vi "final result simple.vi"(4 "norm type":string="std norm", 6 "q":string="17O q", 9 "error in":errorcluster) -> (1 "error out":errorcluster)   [LabVIEW 2016]
uses:
  <vilib>/Analysis/baseanly.llb/Mean (DBL).vi
  <vilib>/Analysis/NI_AALBase.lvlib
panel:
  out "array w/ subset deleted 2":dbl[][](array[numeric])
  out "size(s)":i32
  out "array w/ subset deleted":dbl[][](array[numeric])
  out "Numeric 4":i32
  out "Numeric 3":i32
  out "Numeric 2":i32
  out "sqrt(x) 3":dbl
  out "sqrt(x) 2":dbl
  out "sqrt(x)":dbl
  out "Array 4":dbl[](array[numeric])
  out "Array 15":dbl[](array[numeric])
  out "Array 14":dbl[](array[numeric])
  out "sequence result header":string[](array[string])
  out "subarray 2":string[](array[string])
  in  "Final result header":string[](array[string])=["position", "holder", "sample name", "number of cycles", "user", "Total Run Time(min)", "final ratio", "error", "percent error"]
  out "Array 13":dbl[](array[numeric])
  out "Array 12":dbl[](array[numeric])
  out "Array 11":dbl[](array[numeric])
  out "Final Result 2":string[][](array[string])
  out "Array 8":dbl[](array[numeric])
  out "Array 7":dbl[](array[numeric])
  out "subarray":dbl[](array[numeric])
  out "Numeric":dbl
  out "Cycle data by seq":dbl[][][](array[numeric])
  out "appended array":dbl[](array[numeric])
  out "Array 3":string[][](array[string])
  out "Array 2":string[](array[string])
  out "Array":string[][](array[string])
  out "sequence  Result":dbl[][](array[numeric])
  out "Final result header 2":string[](array[string])
  out "Final Result":string[](array[string])
  out "cycle result header":string[](array[string])
  out "Array 5":dbl[](array[numeric])
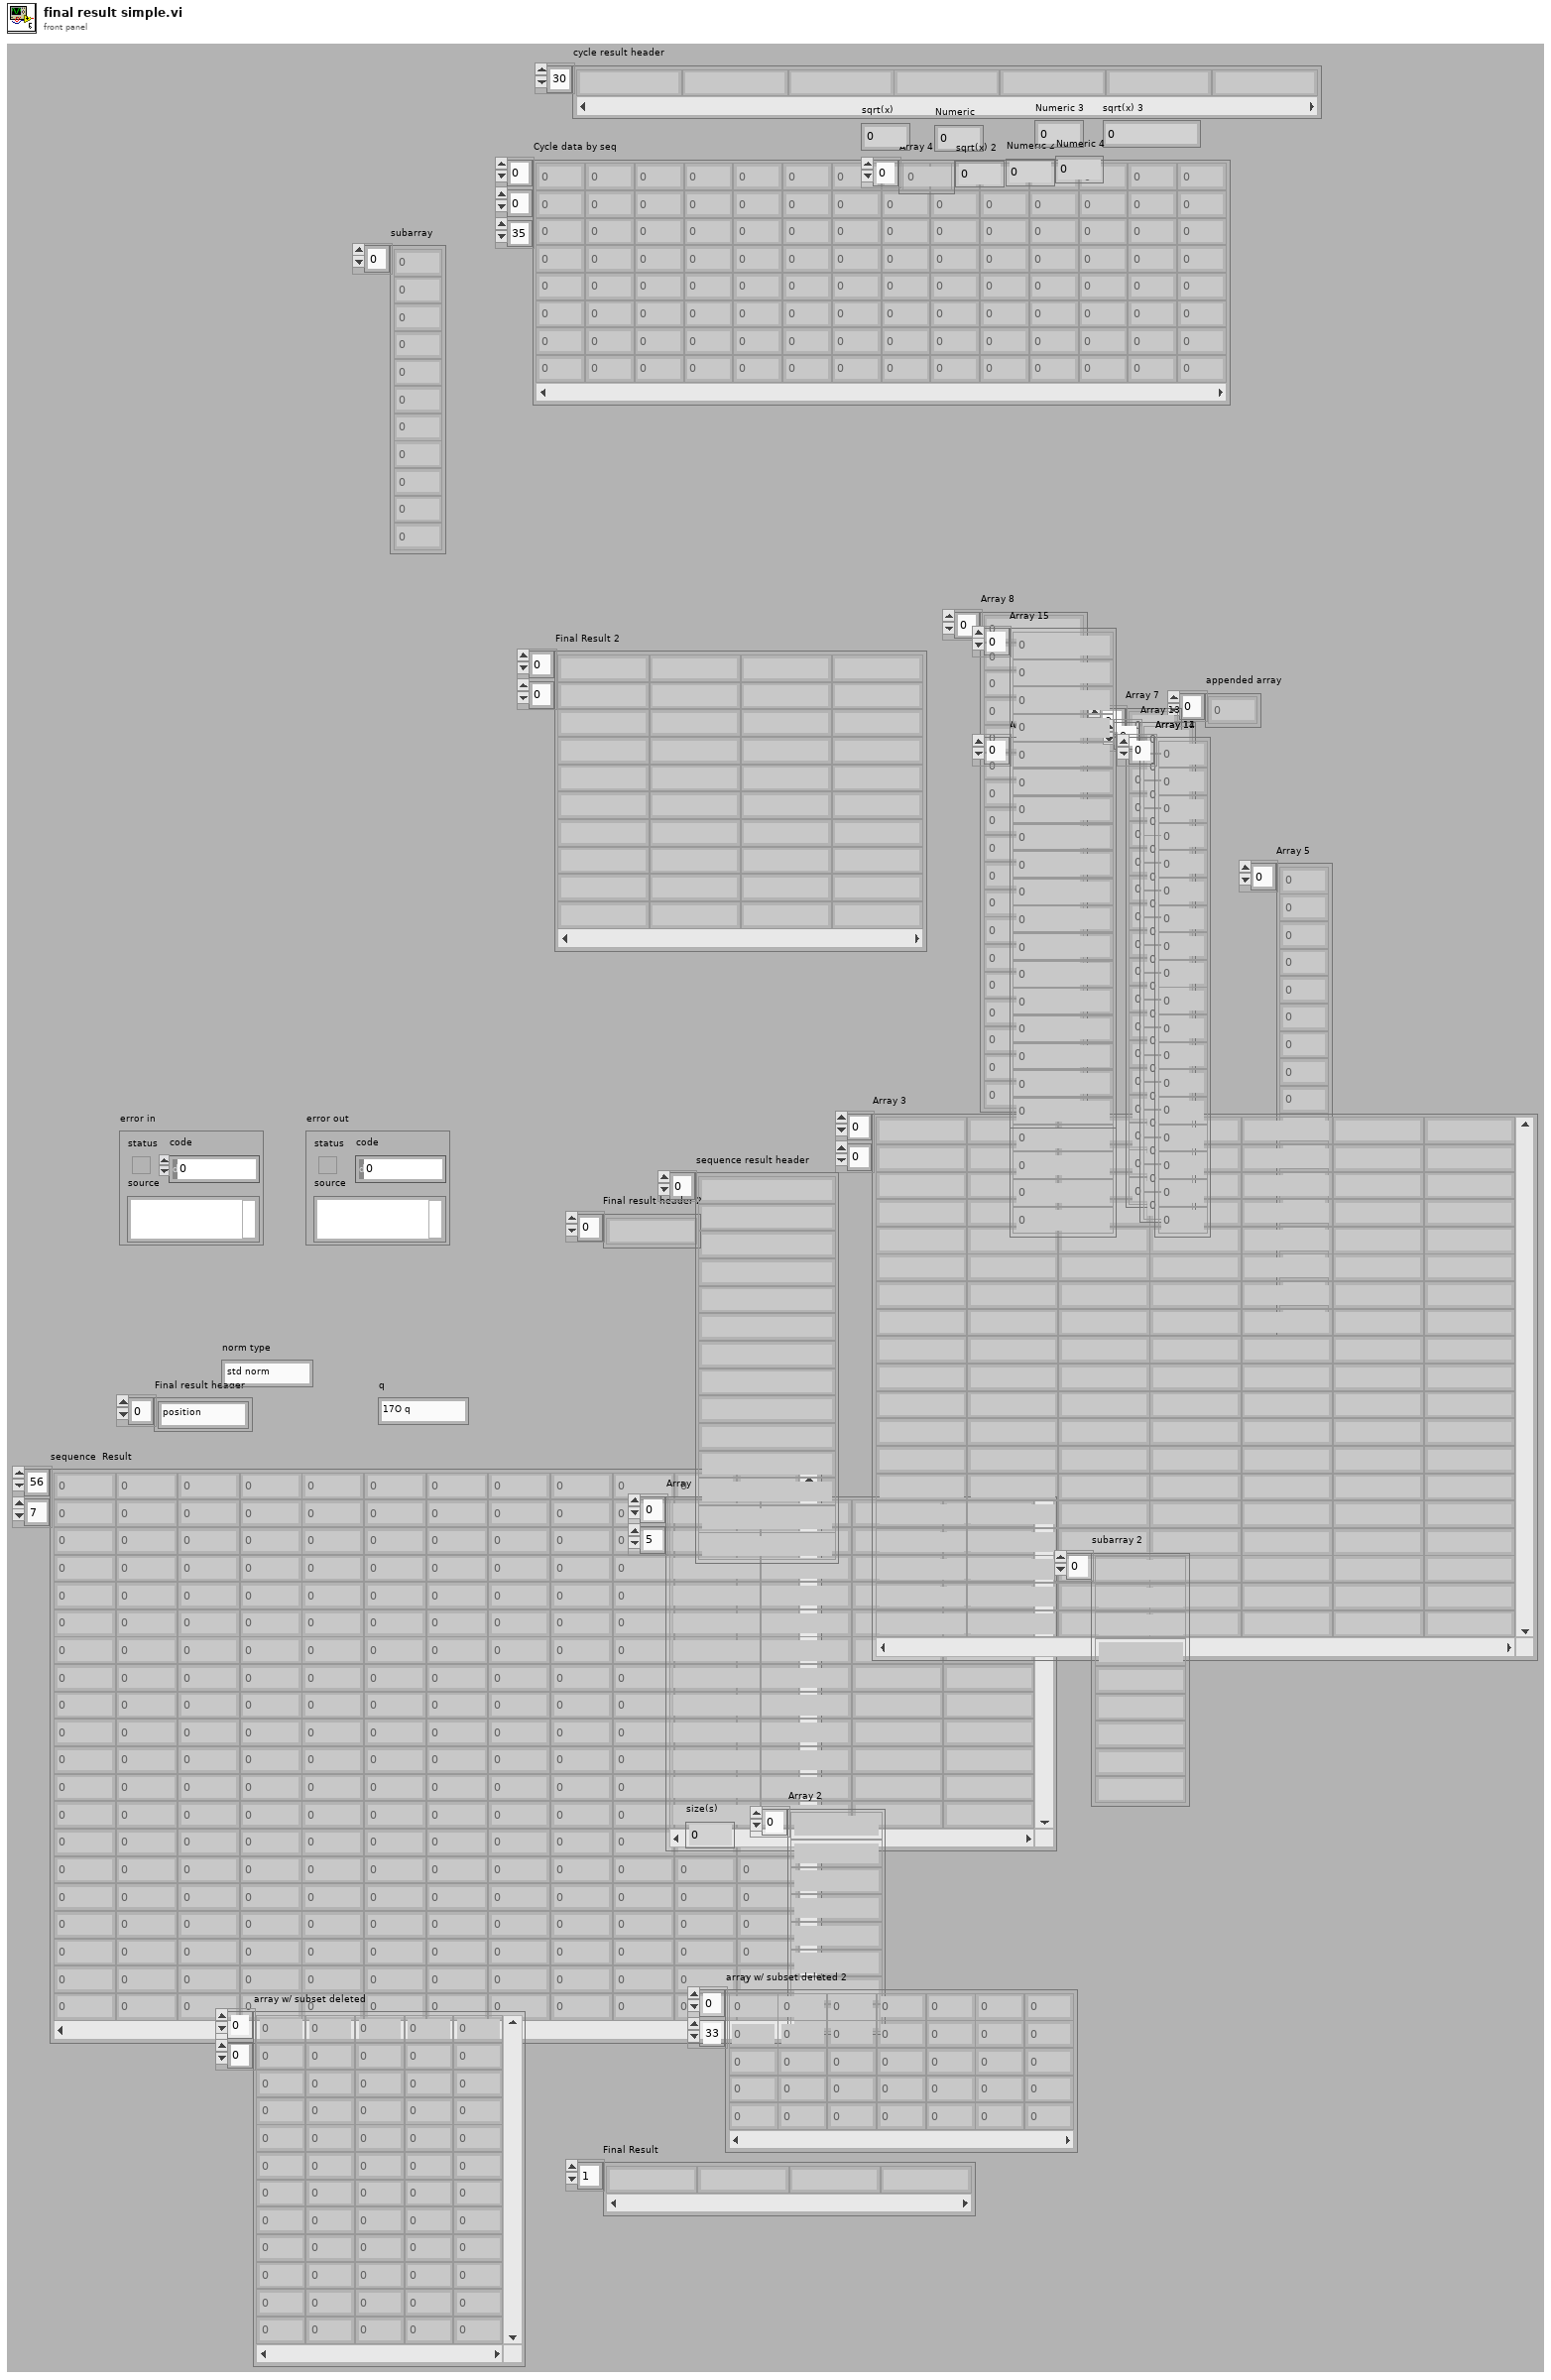
[diagram p1: front panel]
types:
  T1 = typedef "data control cluster.ctl" = cluster{"Final result header":string[], "sequence result header":string[], "cycle result header ":string[], "Final Result":string[][], "sequence  Result":dbl[][], "Cycle data by seq":dbl[][][], "Cycle data by position":dbl[][][], "Final seq  Result":dbl[][], "only specific type":dbl[][]}
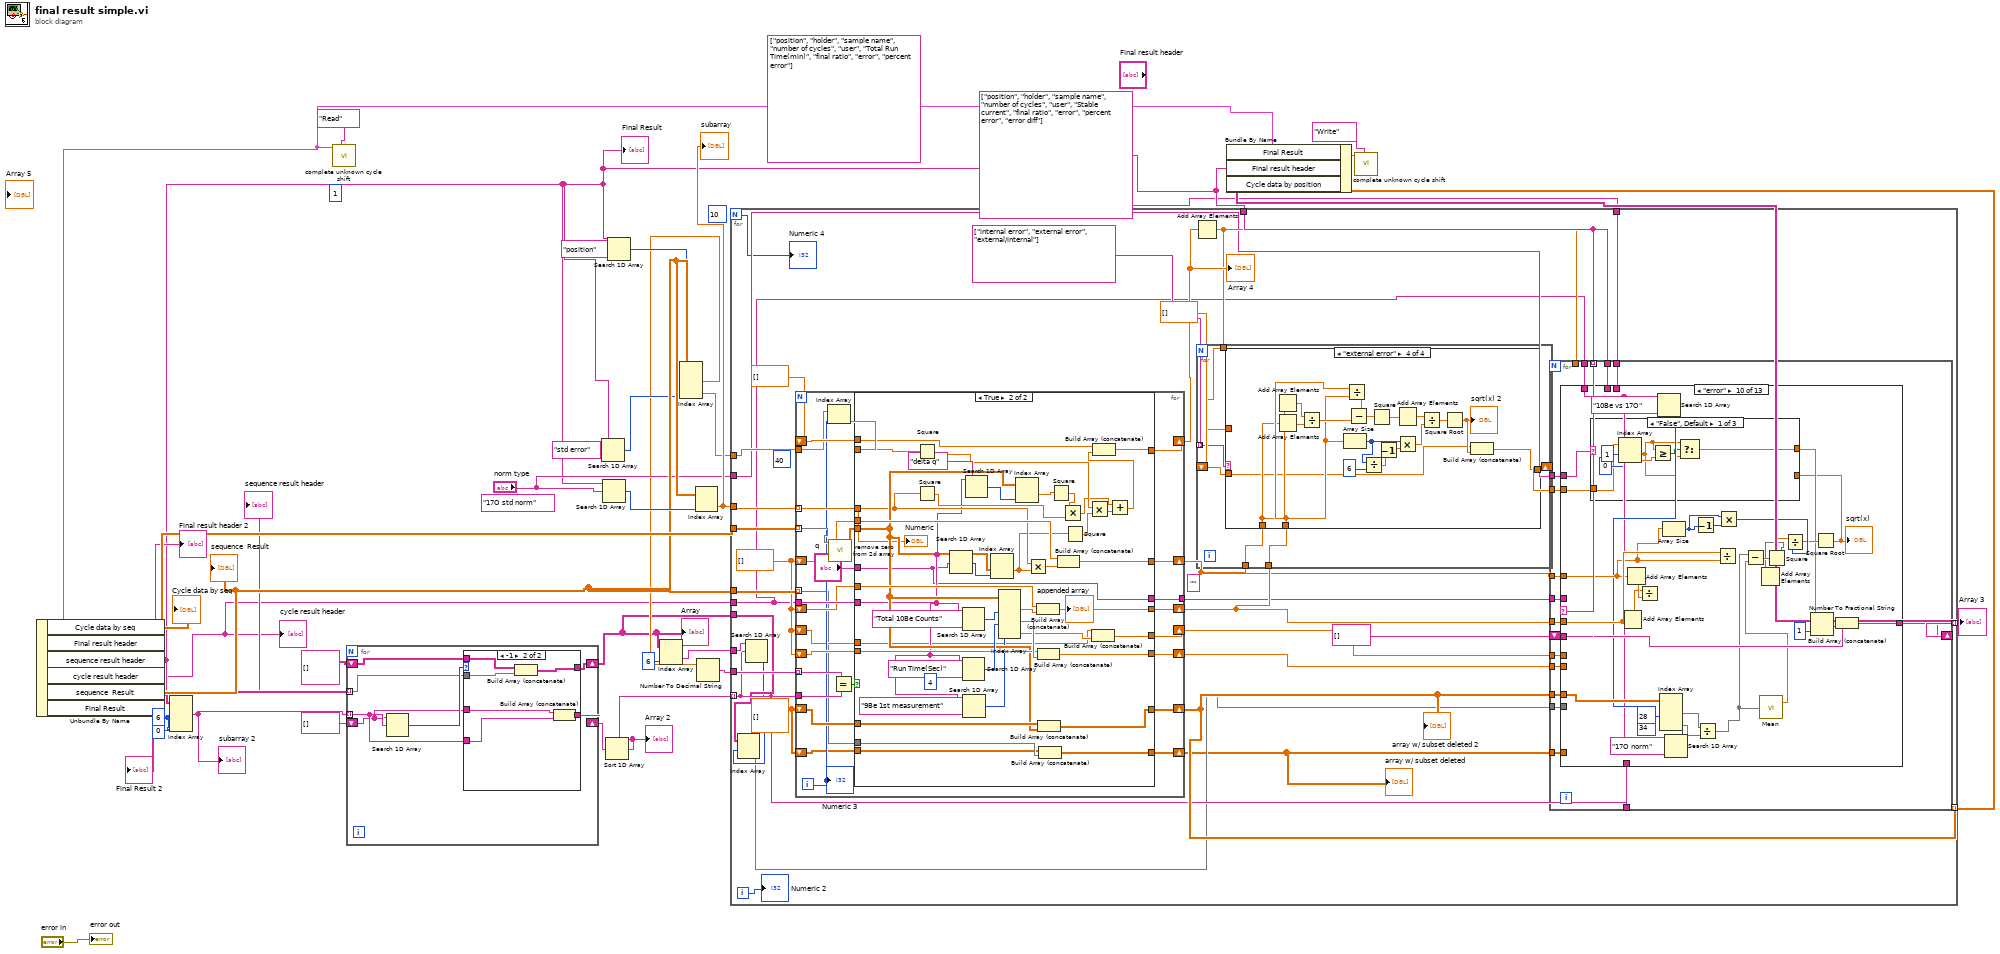
[diagram p0: block diagram]
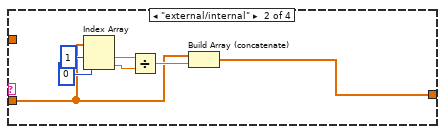
[diagram p3: hidden frame]
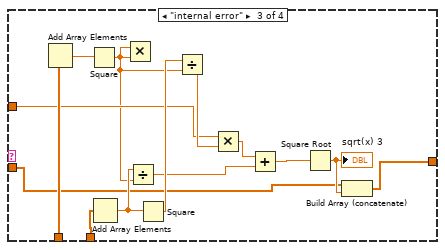
[diagram p4: hidden frame]
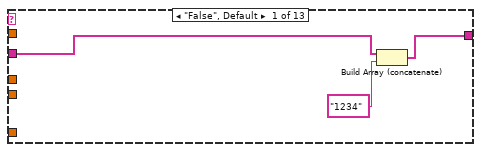
[diagram p5: hidden frame]
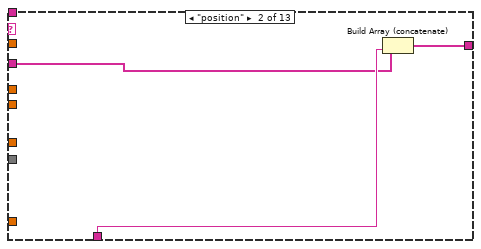
[diagram p6: hidden frame]
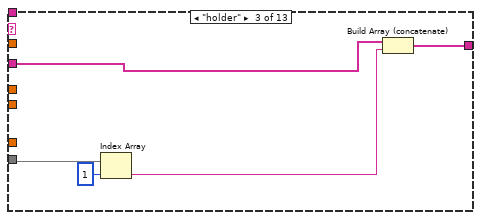
[diagram p7: hidden frame]
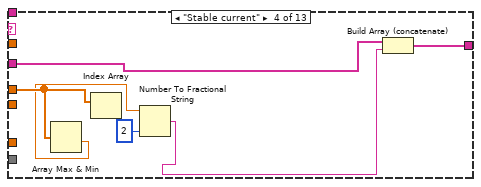
[diagram p8: hidden frame]
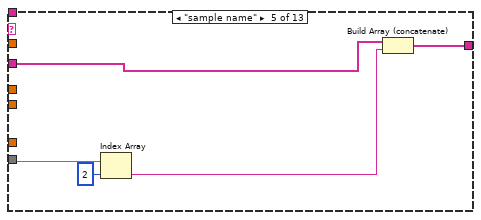
[diagram p9: hidden frame]
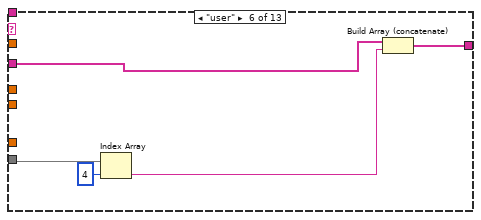
[diagram p10: hidden frame]
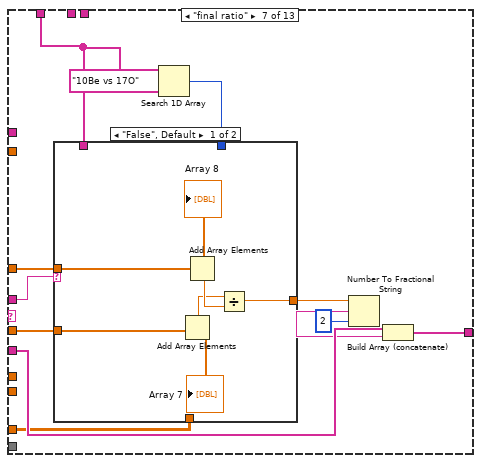
[diagram p11: hidden frame]
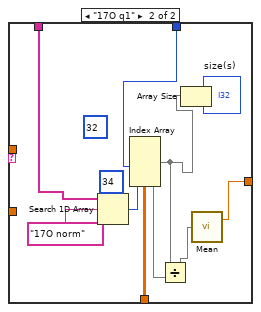
[diagram p12: hidden frame]
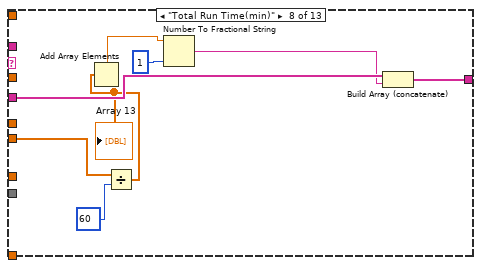
[diagram p13: hidden frame]
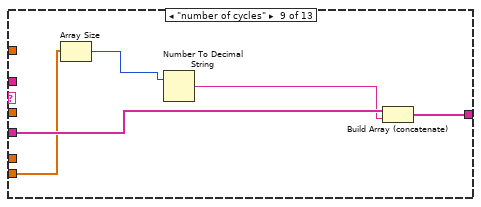
[diagram p14: hidden frame]
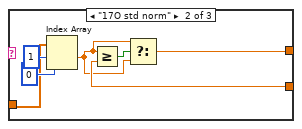
[diagram p15: hidden frame]
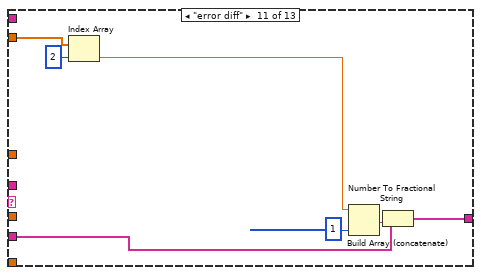
[diagram p17: hidden frame]
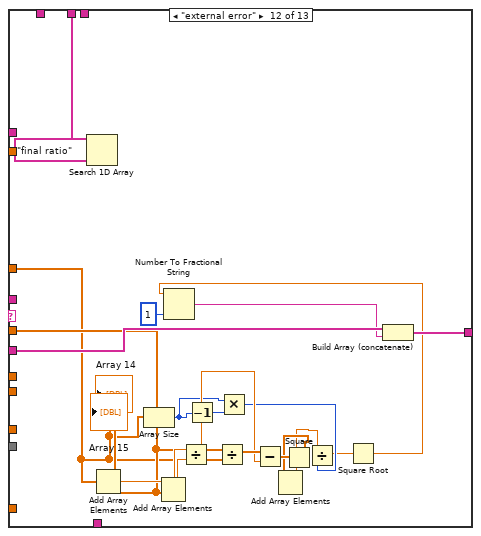
[diagram p18: hidden frame]
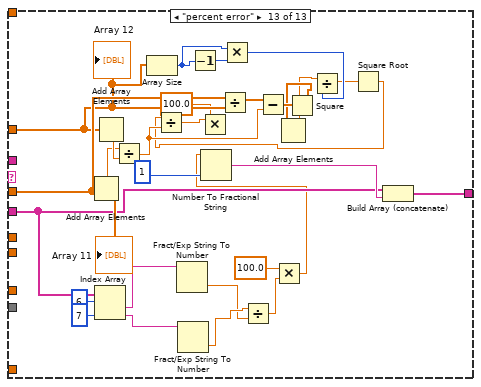
[diagram p19: hidden frame]
diagram:
  (unwired) "17O std norm" ("element")
  w14 = string[] ["position", "holder", "sample name", "number of cycles", "user", "Stable current", "final ratio", "error", "percent error", "error diff"] ("Final result header")
  (unwired) string[] ["position", "holder", "sample name", "number of cycles", "user", "Total Run Time(min)", "final ratio", "error", "percent error"] ("Final result header")
  (unwired) 10
  w28 = 6 ("disabled index (col)")
  (unwired) 1
  n1 = call "complete unknown cycle shift.vi"("read write shift"="Read") -> ("DATA CLUSTER out"=w18:T1)  [unwired: 9 in, 1 out]
  n2 = Unbundle By Name(w18) -> ("Cycle data by seq"=w25:dbl[][][], "Final result header"=→"Final result header 2":string[], "sequence result header"=w2:string[], "cycle result header"=w1:string[], "sequence  Result"=w16:dbl[][], "Final Result"=w13:string[][])
  "cycle result header" <- w1
  "Final Result" <- w2
  "sequence  Result" <- w16
  "Cycle data by seq" <- w25
  "Final Result 2" <- w13
  "sequence result header" <- w2
  n3 = Index Array(array=w13, index (col) #1=w28, index (row) #2=0 ("disabled index (row)"), index (col) #2=w28) -> (element #1=w30:string[])  [unwired: 1 in, 1 out]
  "subarray 2" <- w30
  n4 = for {
    tunnel: w30 -> [w37] mode=indexing
    tunnel: w13 -> [w40] mode=indexing
    shift-right: [w39] -> w5
    shift-left: string[][] [] -> [w38]
    shift-right: [w36] -> w8
    shift-left: string[] [] -> [w35]
    n5 = Search 1D Array(1D array=w35, element=w37) -> (index of element=w41:i32)  [unwired: 1 in]
    n6 = case shown="-1" w41 {
      tunnel: w40 -> [_ w49]
      tunnel: [w43 w48] -> w39
      tunnel: w38 -> [w43 w47]
      tunnel: w37 -> [_ w46]
      tunnel: [w42 w45] -> w36
      tunnel: w35 -> [w42 w44]
      frame 0, Default {
      }
      frame -1 {
        n7 = Build Array (concatenate)(w47, w49) -> (w48:string[][])
        n8 = Build Array (concatenate)(w44, w46) -> (w45:string[])
      }
    }
  }
  "Array" <- w5
  n9 = Search 1D Array(1D array=w2, element="std error") -> (index of element=w11:i32)  [unwired: 1 in]
  n10 = Search 1D Array(1D array=w2, element="norm type") -> (index of element=w23:i32)  [unwired: 1 in]
  n11 = Sort 1D Array(array=w8) -> (sorted array=w7:string[])
  "Array 2" <- w7
  n12 = Search 1D Array(1D array=w2, element="position") -> (index of element=w15:i32)  [unwired: 1 in]
  n13 = Index Array(array=w5, index (col)=6 ("disabled index (col)")) -> (element=w3:string[])  [unwired: 1 in]
  n14 = Index Array(array=w16, index (col) #1=w15, index (col) #2=w11) -> (element #1=w6:dbl[], element #2=w10:dbl[])  [unwired: 2 in]
  n15 = Index Array(array=w16, index (col)=w23) -> (element=w22:dbl[])  [unwired: 1 in]
  "subarray" <- w22
  n16 = Number To Decimal String(number=w6) -> (decimal integer string=w24:string[])  [unwired: 1 in]
  n17 = for {
    N -> [w62]
    tunnel: w7 -> [w58] mode=indexing
    tunnel: w16 -> [w82]
    tunnel: w25 -> [w78]
    tunnel: w24 -> [w80]
    tunnel: w22 -> [w81]
    tunnel: w1 -> [w50]
    tunnel: [w79] -> w20 mode=indexing
    tunnel: w14 -> [w74]
    tunnel: w5 -> [w57]
    tunnel: [w75] -> w17 mode=indexing
    tunnel: w10 -> [w73]
    tunnel: "norm type" -> [w64]
    tunnel: w3 -> [w59]
    tunnel: w2 -> [w54]
    i -> [w63]
    w53 = dbl[][] [] ("array w/ subset deleted")
    (unwired) "" ("String")
    (unwired) 40
    w60 = dbl[] []
    n18 = Search 1D Array(1D array=w59, element=w58) -> (index of element=w56:i32)  [unwired: 1 in]
    n19 = Index Array(array=w57, index (row)=w56) -> (element=w55:string[])  [unwired: 1 in]
    n20 = for {
      tunnel: w78 -> [w331] mode=indexing
      tunnel: w82 -> [w318] mode=indexing
      tunnel: w80 -> [w338] mode=indexing
      tunnel: w58 -> [w339]
      tunnel: w81 -> [w336] mode=indexing
      tunnel: w50 -> [w335]
      shift-right: [w334] -> w68
      shift-left: w60 -> [w333]
      shift-right: [w330] -> w67
      shift-left: w60 -> [w332]
      shift-right: [w329] -> w76
      shift-left: w60 -> [w328]
      shift-right: [w327] -> w75
      shift-left: w53 -> [w326]
      tunnel: w73 -> [w323]
      shift-right: [w325] -> w71
      shift-left: dbl[] [] -> [w324]
      shift-right: [w320] -> w61
      shift-left: w60 -> [w319]
      shift-right: [w317] -> w52
      shift-left: w53 -> [w316]
      tunnel: [w315] -> w51
      i -> [w322]
      n21 = Index Array(array=w323, index=w322) -> (element=w321:dbl)
      n22 = call "remove zero from 2d array.vi"("Cycle data by seq"=w331) -> ("array w/ subset deleted"=w313:dbl[][])  [unwired: 10 in]
      n23 = Equal?(x=w338, y=w339) -> (x = y?=w337:bool)
      n24 = case shown="True" w337 {
        tunnel: w336 -> [_ w366]
        tunnel: w313 -> [_ w368]
        tunnel: w335 -> [_ w356]
        tunnel: [w346 w384] -> w334
        tunnel: w333 -> [w346 w383]
        tunnel: [w347 w382] -> w330
        tunnel: w332 -> [w347 w381]
        tunnel: [w345 w378] -> w329
        tunnel: w328 -> [w345 w376]
        tunnel: [w344 w375] -> w327
        tunnel: w326 -> [w344 w374]
        tunnel: w321 -> [_ w373]
        tunnel: [w343 w358] -> w325
        tunnel: w324 -> [w343 w372]
        tunnel: [w342 w353] -> w320
        tunnel: w319 -> [w342 w352]
        tunnel: w318 -> [_ w351]
        tunnel: [w341 w350] -> w317
        tunnel: w316 -> [w341 w349]
        tunnel: [w340 w348] -> w315
        tunnel: "q" -> [w340 w348]
        frame False {
        }
        frame True {
          (unwired) 4 ("index (col)")
          n25 = Square(x=w373) -> (x^2=w362:dbl)
          n26 = Square(x=w366) -> (x^2=w365:dbl)
          n27 = Search 1D Array(1D array=w356, element=w348) -> (index of element=w386:i32)  [unwired: 1 in]
          n28 = Search 1D Array(1D array=w356, element="Total 10Be Counts") -> (index of element=w388:i32)  [unwired: 1 in]
          n29 = Search 1D Array(1D array=w356, element="Run Time(Sec)") -> (index of element=w379:i32)  [unwired: 1 in]
          n30 = Search 1D Array(1D array=w356, element="9Be 1st measurement") -> (index of element=w355:i32)  [unwired: 1 in]
          n31 = Search 1D Array(1D array=w356, element="delta q" ("q 2")) -> (index of element=w371:i32)  [unwired: 1 in]
          n32 = Index Array(array=w368, index (col)=w386) -> (element=w364:dbl[])  [unwired: 1 in]
          n33 = Index Array(array=w368, index (col) #1=w388, index (col) #2=w379, index (col) #3=w355) -> (element #1=w387:dbl[], element #2=w377:dbl[], element #3=w354:dbl[])  [unwired: 3 in]
          n34 = Index Array(array=w368, index (col)=w371) -> (element=w369:dbl[])  [unwired: 1 in]
          n35 = Multiply(x=w366, y=w364) -> (x*y=w385:dbl[])
          n36 = Build Array (concatenate)(w383, w387) -> (w384:dbl[])
          "appended array" <- w384
          n37 = Build Array (concatenate)(w376, w377) -> (w378:dbl[])
          n38 = Build Array (concatenate)(w374, w368) -> (w375:dbl[][])
          n39 = Build Array (concatenate)(w349, w351) -> (w350:dbl[][])
          n40 = Square(x=w369) -> (x^2=w367:dbl[])
          n41 = Build Array (concatenate)(w381, w385) -> (w382:dbl[])
          n42 = Multiply(x=w367, y=w365) -> (x*y=w360:dbl[])
          n43 = Square(x=w364) -> (x^2=w363:dbl[])
          n44 = Multiply(x=w362, y=w363) -> (x*y=w361:dbl[])
          n45 = Build Array (concatenate)(w352, w354) -> (w353:dbl[])
          n46 = Add(x=w360, y=w361) -> (x+y=w359:dbl[])
          n47 = Build Array (concatenate)(w372, w359) -> (w358:dbl[])
          "Numeric" <- w366
        }
      }
      "Numeric 3" <- w322
    }
    "Array 4" <- w71
    "array w/ subset deleted" <- w52
    "array w/ subset deleted 2" <- w75
    n48 = Add Array Elements(numeric array=w71) -> (sum=w69:dbl)
    n49 = for {
      tunnel: string[] ["internal error", "external error", "external/internal"] -> [w88] mode=indexing
      tunnel: w69 -> [w87]
      tunnel: w68 -> [w86]
      tunnel: w67 -> [w85]
      shift-right: [w84] -> w65
      shift-left: dbl[] [] -> [w83]
      n50 = case shown="\"external error\"" w88 {
        tunnel: w87 -> [_ _ w104 _]
        tunnel: w86 -> [_ _ w110 w118]
        tunnel: w85 -> [_ _ w109 w117]
        tunnel: [w89 w90 w99 w116] -> w84
        tunnel: w83 -> [w89 w91 w98 w114]
        frame "False", Default {
        }
        frame "external/internal" {
          n51 = Index Array(array=w91, index #1=1 ("index"), index #2=0 ("index")) -> (element #1=w93:dbl, element #2=w94:dbl)
          n52 = Divide(x=w93, y=w94) -> (x/y=w92:dbl)
          n53 = Build Array (concatenate)(w91, w92) -> (w90:dbl[])
        }
        frame "internal error" {
          n54 = Add Array Elements(numeric array=w109) -> (sum=w108:dbl)
          n55 = Square(x=w108) -> (x^2=w97:dbl)
          n56 = Add Array Elements(numeric array=w110) -> (sum=w107:dbl)
          n57 = Multiply(x=w97, y=w97) -> ()  [unwired: 1 out]
          n58 = Divide(x=w107, y=w97) -> (x/y=w102:dbl)
          n59 = Square(x=w107) -> (x^2=w106:dbl)
          n60 = Divide(x=w106, y=w97) -> (x/y=w105:dbl)
          n61 = Multiply(x=w104, y=w105) -> (x*y=w103:dbl)
          n62 = Add(x=w103, y=w102) -> (x+y=w101:dbl)
          n63 = Square Root(x=w101) -> (sqrt(x)=w100:dbl)
          "sqrt(x) 3" <- w100
          n64 = Build Array (concatenate)(w98, w100) -> (w99:dbl[])
        }
        frame "external error" {
          n65 = Add Array Elements(numeric array=w118) -> (sum=w127:dbl)
          n66 = Add Array Elements(numeric array=w117) -> (sum=w128:dbl)
          n67 = Divide(x=w127, y=w128) -> (x/y=w125:dbl)
          n68 = Array Size(array=w117) -> (size(s)=w113:i32)
          n69 = Divide(x=w118, y=w117) -> (x/y=w126:dbl[])
          n70 = Subtract(x=w126, y=w125) -> (x-y=w124:dbl[])
          n71 = Divide(x=w113, y=6) -> (x/y=w111:dbl)
          n72 = Square(x=w124) -> (x^2=w120:dbl[])
          n73 = Decrement(x=w111) -> (x-1=w123:dbl)
          n74 = Add Array Elements(numeric array=w120) -> (sum=w119:dbl)
          n75 = Multiply(x=w113, y=w123) -> (x*y=w122:dbl)
          n76 = Divide(x=w119, y=w122) -> (x/y=w121:dbl)
          n77 = Square Root(x=w121) -> (sqrt(x)=w115:dbl)
          "sqrt(x) 2" <- w115
          n78 = Build Array (concatenate)(w114, w115) -> (w116:dbl[])
        }
      }
    }
    n79 = for {
      tunnel: w68 -> [w145]
      tunnel: w58 -> [w144]
      tunnel: w67 -> [w143]
      tunnel: w74 -> [w142] mode=indexing
      shift-right: [w140] -> w79
      shift-left: string[] [] -> [w141]
      tunnel: w55 -> [w139]
      tunnel: w76 -> [w138]
      tunnel: w75 -> [w137]
      tunnel: w74 -> [w136]
      tunnel: w69 -> [_]
      tunnel: w65 -> [w135]
      tunnel: w64 -> [w134]
      tunnel: w61 -> [w133]
      tunnel: w54 -> [w130]
      tunnel: w52 -> [w132]
      tunnel: w51 -> [w131]
      tunnel: w50 -> [w129]
      n80 = case shown="\"error\"" w142 {
        tunnel: w145 -> [_ _ _ _ _ _ w184 _ _ w236 _ w278 w308]
        tunnel: w144 -> [_ w151 _ _ _ _ _ _ _ _ _ _ _]
        tunnel: w143 -> [_ _ _ _ _ _ w182 _ _ w234 _ w274 w305]
        tunnel: w141 -> [w147 w150 w156 w162 w167 w172 w181 w207 w212 w239 w263 w281 w293]
        tunnel: [w146 w149 w155 w161 w166 w171 w180 w206 w211 w238 w262 w280 w310] -> w140
        tunnel: w139 -> [_ _ w154 _ w165 w170 _ _ _ _ _ _ _]
        tunnel: w138 -> [_ _ _ _ _ _ _ w204 w209 _ _ _ _]
        tunnel: w137 -> [_ _ _ _ _ _ w174 _ _ w220 _ _ _]
        tunnel: w136 -> [_ _ _ _ _ _ _ _ _ _ _ w265 _]
        tunnel: w135 -> [_ _ _ _ _ _ _ _ _ w226 w258 _ _]
        tunnel: w134 -> [_ _ _ _ _ _ _ _ _ w224 _ _ _]
        tunnel: w133 -> [_ _ _ w158 _ _ _ _ _ _ _ _ _]
        tunnel: w132 -> [_ _ _ _ _ _ _ _ _ _ _ _ _]
        tunnel: w131 -> [_ _ _ _ _ _ w176 _ _ _ _ _ _]
        tunnel: w130 -> [_ _ _ _ _ _ _ _ _ _ _ _ _]
        tunnel: w129 -> [_ _ _ _ _ _ w173 _ _ w214 _ _ _]
        frame "False", Default {
          n81 = Build Array (concatenate)(w147, "1234" ("String")) -> (w146:string[])
        }
        frame "position" {
          n82 = Build Array (concatenate)(w150, w151) -> (w149:string[])
        }
        frame "holder" {
          n83 = Index Array(array=w154, index=1) -> (element=w152:string)
          n84 = Build Array (concatenate)(w156, w152) -> (w155:string[])
        }
        frame "Stable current" {
          n85 = Array Max & Min(array=w158) -> (min value=w157:dbl)  [unwired: 3 out]
          n86 = Index Array(array=w158) -> ()  [unwired: 1 in, 1 out]
          n87 = Number To Fractional String(number=w157, precision (6)=i16 2) -> (F-format string=w159:string)  [unwired: 2 in]
          n88 = Build Array (concatenate)(w162, w159) -> (w161:string[])
        }
        frame "sample name" {
          n89 = Index Array(array=w165, index=2) -> (element=w163:string)
          n90 = Build Array (concatenate)(w167, w163) -> (w166:string[])
        }
        frame "user" {
          n91 = Index Array(array=w170, index=4) -> (element=w168:string)
          n92 = Build Array (concatenate)(w172, w168) -> (w171:string[])
        }
        frame "final ratio" {
          n93 = Search 1D Array(1D array=w173, element="10Be vs 17O") -> (index of element=w175:i32)  [unwired: 1 in]
          n94 = case shown="\"False\", Default" w176 {
            tunnel: w184 -> [w188 _]
            tunnel: [w187 w198] -> w183
            tunnel: w182 -> [w186 _]
            tunnel: w175 -> [_ w193]
            tunnel: w174 -> [_ w199]
            tunnel: w173 -> [_ w191]
            frame "False", Default {
              n95 = Add Array Elements(numeric array=w188) -> (sum=w185:dbl)
              n96 = Add Array Elements(numeric array=w186) -> (sum=w189:dbl)
              n97 = Divide(x=w185, y=w189) -> (x/y=w187:dbl)
              "Array 8" <- w186
              "Array 7" <- w188
            }
            frame "17O q1" {
              (unwired) 32 ("disabled index (col)")
              (unwired) 34 ("index (col)")
              n98 = Search 1D Array(1D array=w191, element="17O norm") -> (index of element=w190:i32)  [unwired: 1 in]
              n99 = Index Array(array=w199, index (col) #1=w193, index (col) #2=w190) -> (element #1=w196:dbl[], element #2=w195:dbl[])  [unwired: 2 in]
              n100 = Divide(x=w196, y=w195) -> (x/y=w194:dbl[])
              n101 = Array Size(array=w196) -> (size(s)=→"size(s)":i32)
              n102 = call-poly <vilib>:"Mean.vi"("X"=w194) -> ("mean"=w198:dbl)  [unwired: 1 out]
            }
          }
          n103 = Number To Fractional String(number=w183, precision (6)=i16 2) -> (F-format string=w179:string)  [unwired: 2 in]
          n104 = Build Array (concatenate)(w181, w179) -> (w180:string[])
        }
        frame "Total Run Time(min)" {
          n105 = Divide(x=w204, y=60 ("Numeric")) -> (x/y=w202:dbl[])
          "Array 13" <- w202
          n106 = Add Array Elements(numeric array=w202) -> (sum=w201:dbl)
          n107 = Number To Fractional String(number=w201, precision (6)=i16 1) -> (F-format string=w205:string)  [unwired: 2 in]
          n108 = Build Array (concatenate)(w207, w205) -> (w206:string[])
        }
        frame "number of cycles" {
          n109 = Array Size(array=w209) -> (size(s)=w208:i32)
          n110 = Number To Decimal String(number=w208) -> (decimal integer string=w210:string)  [unwired: 1 in]
          n111 = Build Array (concatenate)(w212, w210) -> (w211:string[])
        }
        frame "error" {
          (unwired) 34 ("index (col)")
          (unwired) 28 ("disabled index (col)")
          n112 = Add Array Elements(numeric array=w236) -> (sum=w240:dbl)
          n113 = Add Array Elements(numeric array=w234) -> (sum=w241:dbl)
          n114 = Divide(x=w240, y=w241) -> ()  [unwired: 1 out]
          n115 = Search 1D Array(1D array=w214, element="10Be vs 17O") -> (index of element=w216:i32)  [unwired: 1 in]
          n116 = Array Size(array=w234) -> (size(s)=w232:i32)
          n117 = Search 1D Array(1D array=w214, element="17O norm") -> (index of element=w213:i32)  [unwired: 1 in]
          n118 = Index Array(array=w220, index (col) #1=w216, index (col) #2=w213) -> (element #1=w218:dbl[], element #2=w219:dbl[])  [unwired: 2 in]
          n119 = Decrement(x=w232) -> (x-1=w233:i32)
          n120 = Divide(x=w218, y=w219) -> (x/y=w217:dbl[])
          n121 = Divide(x=w236, y=w234) -> ()  [unwired: 1 out]
          n122 = Multiply(x=w232, y=w233) -> (x*y=w231:i32)
          n123 = call-poly <vilib>:"Mean.vi"("X"=w217) -> ("mean"=w221:dbl)  [unwired: 1 out]
          n124 = Subtract(x=w217, y=w221) -> (x-y=w235:dbl[])
          n125 = Square(x=w235) -> (x^2=w229:dbl[])
          n126 = Add Array Elements(numeric array=w229) -> (sum=w228:dbl)
          n127 = Divide(x=w228, y=w231) -> (x/y=w230:dbl)
          n128 = Square Root(x=w230) -> (sqrt(x)=w223:dbl)
          "sqrt(x)" <- w223
          n129 = case shown="\"False\", Default" w224 {
            tunnel: w226 -> [w246 w253 _]
            tunnel: [w243 w251 w256] -> w225
            tunnel: w223 -> [_ w250 w256]
            frame "False", Default {
              n130 = Index Array(array=w246, index #1=1 ("index"), index #2=0 ("index")) -> (element #1=w242:dbl, element #2=w244:dbl)
              n131 = Greater Or Equal?(x=w242, y=w244) -> (x >= y?=w245:bool)
              n132 = Select(t=w242, s=w245, f=w242) -> (s? t:f=w243:dbl)
            }
            frame "17O std norm" {
              n133 = Index Array(array=w253, index #1=1 ("index"), index #2=0 ("index")) -> (element #1=w249:dbl)  [unwired: 1 out]
              n134 = Greater Or Equal?(x=w249, y=w250) -> (x >= y?=w252:bool)
              n135 = Select(t=w249, s=w252, f=w249) -> (s? t:f=w251:dbl)
            }
            frame "e" {
            }
          }
          n136 = Number To Fractional String(number=w225, precision (6)=i16 1) -> (F-format string=w237:string)  [unwired: 2 in]
          n137 = Build Array (concatenate)(w239, w237) -> (w238:string[])
        }
        frame "error diff" {
          n138 = Index Array(array=w258, index=2) -> (element=w257:dbl)
          n139 = Number To Fractional String(number=w257, precision (6)=i16 1) -> (F-format string=w261:string)  [unwired: 2 in]
          n140 = Build Array (concatenate)(w263, w261) -> (w262:string[])
        }
        frame "external error" {
          n141 = Search 1D Array(1D array=w265, element="final ratio") -> ()  [unwired: 1 in, 1 out]
          n142 = Add Array Elements(numeric array=w274) -> (sum=w283:dbl)
          n143 = Array Size(array=w274) -> (size(s)=w272:i32)
          n144 = Add Array Elements(numeric array=w278) -> (sum=w282:dbl)
          n145 = Divide(x=w282, y=w283) -> (x/y=w276:dbl)
          n146 = Decrement(x=w272) -> (x-1=w273:i32)
          n147 = Divide(x=w278, y=w274) -> (x/y=w277:dbl[])
          n148 = Multiply(x=w272, y=w273) -> (x*y=w271:i32)
          n149 = Subtract(x=w277, y=w276) -> (x-y=w275:dbl[])
          n150 = Square(x=w275) -> (x^2=w269:dbl[])
          n151 = Add Array Elements(numeric array=w269) -> (sum=w268:dbl)
          n152 = Divide(x=w268, y=w271) -> (x/y=w270:dbl)
          n153 = Square Root(x=w270) -> (sqrt(x)=w267:dbl)
          n154 = Number To Fractional String(number=w267, precision (6)=i16 1) -> (F-format string=w279:string)  [unwired: 2 in]
          n155 = Build Array (concatenate)(w281, w279) -> (w280:string[])
          "Array 15" <- w274
          "Array 14" <- w278
        }
        frame "percent error" {
          n156 = Add Array Elements(numeric array=w308) -> (sum=w311:dbl)
          n157 = Index Array(array=w293, index #1=6 ("index"), index #2=7 ("index")) -> (element #1=w290:string, element #2=w289:string)
          n158 = Add Array Elements(numeric array=w305) -> (sum=w312:dbl)
          n159 = Divide(x=w311, y=w312) -> (x/y=w298:dbl)
          n160 = Array Size(array=w305) -> (size(s)=w303:i32)
          n161 = Fract/Exp String To Number(string=w290) -> (number=w284:dbl)  [unwired: 3 in, 1 out]
          n162 = Fract/Exp String To Number(string=w289) -> (number=w285:dbl)  [unwired: 3 in, 1 out]
          n163 = Decrement(x=w303) -> (x-1=w304:i32)
          n164 = Divide(x=w308, y=w305) -> (x/y=w307:dbl[])
          n165 = Multiply(x=w303, y=w304) -> (x*y=w302:i32)
          n166 = Divide(x=w285, y=w284) -> (x/y=w288:dbl)
          n167 = Subtract(x=w307, y=w298) -> (x-y=w306:dbl[])
          n168 = Multiply(x=100.0, y=w288) -> (x*y=w286:dbl)
          n169 = Number To Fractional String(number=w286, precision (6)=i16 1) -> (F-format string=w309:string)  [unwired: 2 in]
          n170 = Square(x=w306) -> (x^2=w300:dbl[])
          n171 = Add Array Elements(numeric array=w300) -> (sum=w299:dbl)
          n172 = Divide(x=w299, y=w302) -> (x/y=w301:dbl)
          n173 = Square Root(x=w301) -> (sqrt(x)=w297:dbl)
          n174 = Divide(x=w297, y=w298) -> (x/y=w296:dbl)
          n175 = Multiply(x=w296, y=100.0) -> ()  [unwired: 1 out]
          n176 = Build Array (concatenate)(w293, w309) -> (w310:string[])
          "Array 12" <- w305
          "Array 11" <- w308
        }
      }
    }
    "Numeric 2" <- w63
    "Numeric 4" <- w62
  }
  "Array 3" <- w20
  n177 = Bundle By Name(cluster=w18, "Final Result"=w20, "Final result header"=w14, "Cycle data by position"=w17) -> (w19:T1)
  n178 = call "complete unknown cycle shift.vi"("read write shift"="Write", "DATA CLUSTER in"=w19) -> ()  [unwired: 8 in, 2 out]
  "error out" <- "error in"
